vi "Generate Waveform.vi"(0 "signal configuration":refnum<class "SV Continuous Sweep.lvclass">, 5 "template waveform":waveform(dbl), 9 "samples":i32, 11 "error in (no error)":errorcluster) -> (4 "signal configuration":refnum<class "SV Continuous Sweep.lvclass">, 6 "chirp waveform":waveform(dbl), 10 "samples":i32, 15 "error out":errorcluster)   [LabVIEW 2017, in "SV Continuous Sweep.lvclass"]
uses:
  <vilib>/addons/_NISVFA/_Generation/Signal Generation/SV Continuous Sweep/SV Continuous Sweep.lvclass
  C:/Program Files (x86)/National Instruments/LabVIEW 2017/vi.lib/addons/_NISVFA/_Generation/Signal Generation/SV Signal/SV Signal.lvclass
  <vilib>/addons/_NISVFA/_Generation/Signal Generation/SV Continuous Sweep/SV Continuous Sweep.lvclass/SV Continuous Sweep.ctl
  <vilib>/addons/_NISVFA/_Generation/Signal Generation/SV Signal/sv_Signal State Attribute.ctl
  <vilib>/addons/_NISVFA/_Generation/subVIs/sv_Chirp Settings.ctl
  <vilib>/Analysis/1siggen.llb/Ramp Pattern.vi
  <vilib>/Analysis/1siggen.llb/Ramp Pattern by Samples.vi
  <vilib>/addons/_NISVFA/_Generation/Signal Generation/SV Signal/Read Sample Rate.vi
  <vilib>/addons/_NISVFA/_Generation/Signal Generation/SV Signal/SV Signal.lvclass
  <vilib>/addons/_NISVFA/_Generation/SoundVib_Generation.lvlib
  <vilib>/measure/NI_MABase.lvlib
  <vilib>/Analysis/NI_AALBase.lvlib
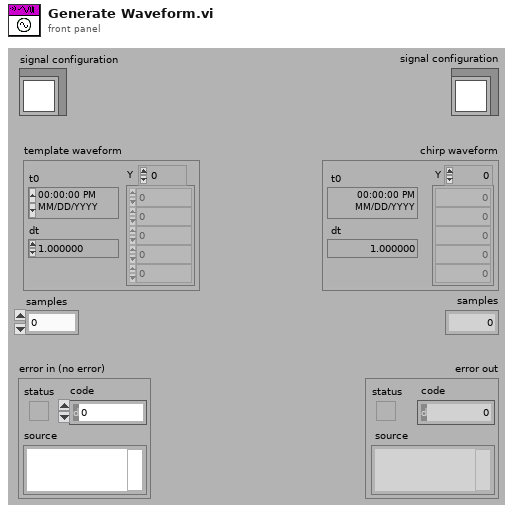
[diagram p1: front panel]
types:
  T1 = cluster{"frequency [Hz]":dbl, "phase [rad]":dbl, "elapsed time [s]":dbl}
  T2 = typedef "SoundVib_Generation.lvlib/sv_Chirp Settings.ctl" = cluster{"amplitude":dbl, "frequency range":cluster{"start (Hz)":dbl, "stop (Hz)":dbl, "frequency spacing":enum16{"Linear", "Logarithmic"}}, "sampling info":cluster{"Fs":dbl, "chirp duration [s]":dbl}, "initial states":cluster{"frequency [Hz]":dbl, "phase [rad]":dbl, "elapsed time [s]":dbl}, "frequency slope":dbl, "maximum harmonic":i32, "prefix len [samples]":cluster{"integer":u32, "fractional":dbl}}
  T3 = typedef "SV Signal.lvclass/sv_System Timing Model.ctl" = i64
  T4 = typedef "SV Signal.lvclass/sv_Generation State.ctl" = enum16{"Idle", "Ramp Up", "Pre-Measurement Settling", "Measurement", "Post-Measurement Settling", "Discrete Sweep Transition", "Ramp Down", "Update"}
  T5 = cluster{"system timing model":T3, "state":cluster{"RESET":bool, "generator timestamp":timestamp, "elapsed seconds":dbl, "elapsed samples":u64, "generation state":T4, "time offset at state":dbl, "samples generated at state":u64, "signal state":variant}, "duration of state":dbl, "samples remaining at state":i32}
  T6 = typedef "SV Signal.lvclass/sv_Signal State Attribute.ctl" = string
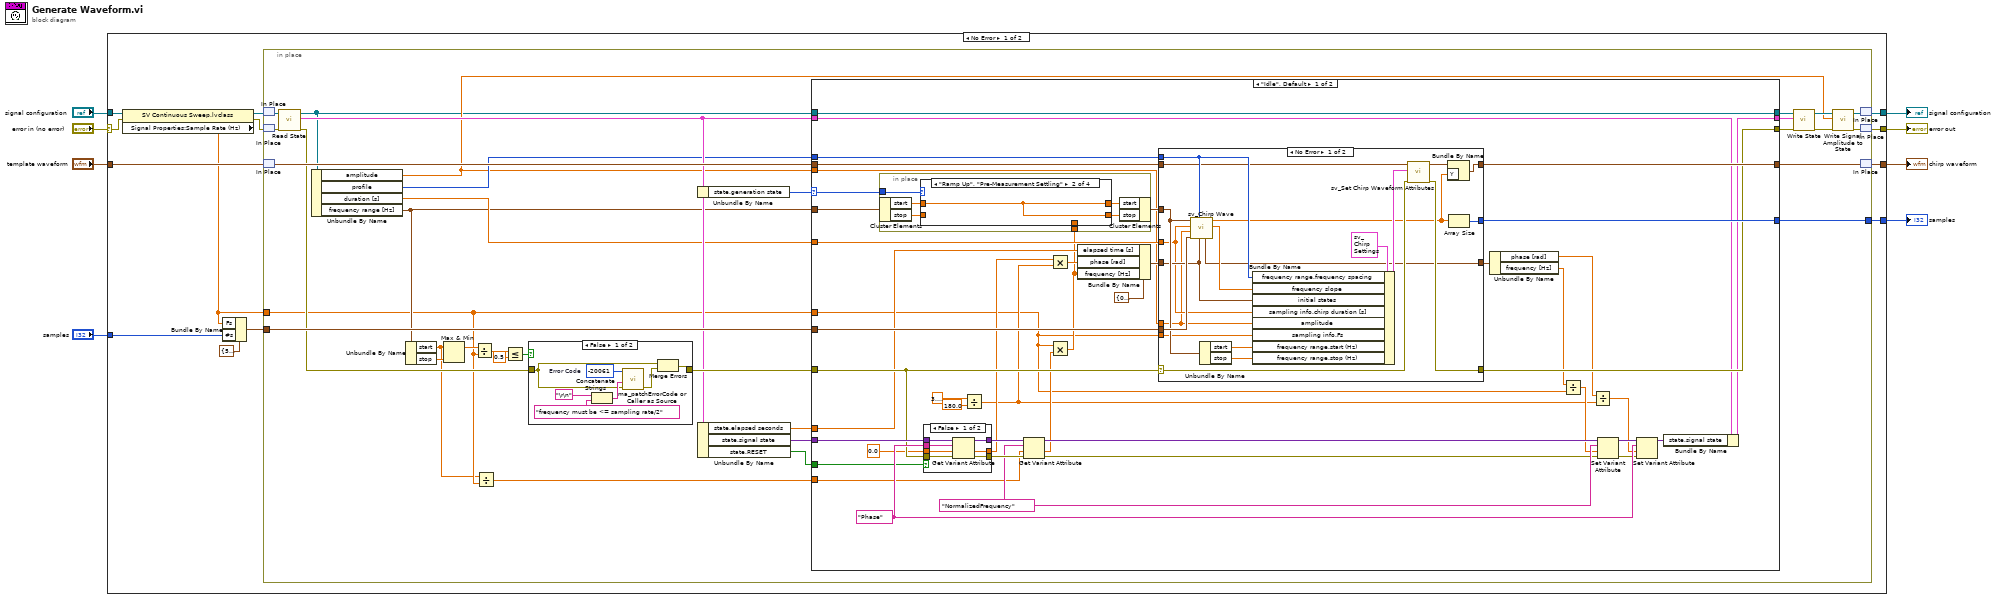
[diagram p0: block diagram]
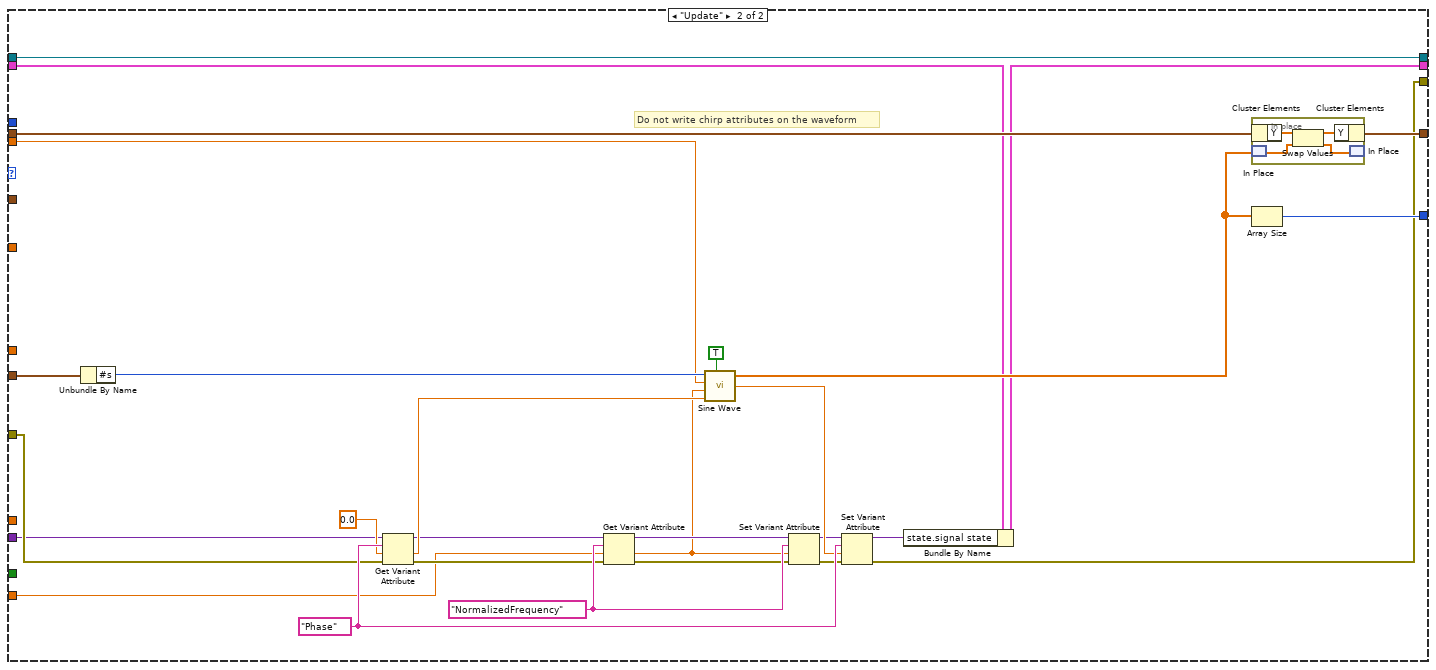
[diagram p7: hidden frame]
diagram:
  n1 = case shown="No Error" "error in (no error)" {
    selector: "error in (no error)" -> [w10 w185]
    tunnel: [w13 w185] -> w7
    tunnel: [w16 w184] -> w5
    tunnel: "signal configuration" -> [w19 w184]
    tunnel: [w14 w183] -> w4
    tunnel: "samples" -> [w20 _]
    tunnel: "template waveform" -> [w15 w183]
    tunnel: [w12 _] -> w1
    frame No Error {
      n2 = property class="SV Continuous Sweep.lvclass"(reference=w19, error in=w10) -> (reference out=w17:refnum<class "SV Continuous Sweep.lvclass">, error out=w9:errorcluster, "Signal Properties:Sample Rate (Hz)"=w11:dbl)
      n3 = Bundle By Name(cluster=cluster{"Fs":dbl, "#s":u32} {"Fs"=51200.0, "#s"=1024} ("sampling info"), "Fs"=w11, "#s"=w20) -> (w18:cluster{"Fs":dbl, "#s":u32})
      n4 = in-place {
        in-place-border: w18 -> [w47]
        in-place-border: [w48] -> w12
        in-place-border: w11 -> [w24]
        n5 = in-place-match #1(w17) -> (w43:refnum<class "SV Continuous Sweep.lvclass">)
        n6 = in-place-match #2(w9) -> (w42:errorcluster)
        n7 = in-place-match #3(w15) -> (w46:waveform(dbl))
        n8 = call <vilib>:"Read State.vi"("error in (no error)"=w42, "signal configuration"=w43) -> ("error out"=w41:errorcluster, "generator state"=w33:T5, "signal configuration"=w27:refnum<class "SV Continuous Sweep.lvclass">)  [unwired: 7 in]
        n9 = Unbundle By Name(w27) -> ("amplitude"=w29:dbl, "profile"=w30:u16, "duration [s]"=w32:dbl, "frequency range [Hz]"=w31:cluster{"start":dbl, "stop":dbl})
        n10 = Unbundle By Name(w31) -> ("start"=w23:dbl, "stop"=w52:dbl)
        n11 = Max & Min(x=w23, y=w52) -> (max(x,y)=w49:dbl)  [unwired: 1 out]
        n12 = Divide(x=w49, y=w24) -> (x/y=w51:dbl)
        n13 = Divide(x=w23, y=w24) -> (x/y=w22:dbl)
        n14 = Less Or Equal?(x=w51, y=0.5) -> (x <= y?=w35:bool)
        n15 = case shown="False" w35 {
          tunnel: [w175 w182] -> w40
          tunnel: w41 -> [w177 w182]
          frame False {
            w178 = -20061  # Error Code
            n16 = Concatenate Strings("\r\n", "frequency must be <= sampling rate/2" ("freq error message")) -> (w181:string)
            n17 = call <vilib>:"ma_patchErrorCode or Caller as Source.vi"("error in (no error)"=w177, "string to append to source"=w181, "error code"=w178) -> ("error out"=w176:errorcluster)  [unwired: 8 in]
            n18 = Merge Errors(w177, w176) -> (w175:errorcluster)
          }
          frame True {
          }
        }
        n19 = Unbundle By Name(w33) -> ("state.generation state"=w28:T4)
        n20 = Unbundle By Name(w33) -> ("state.elapsed seconds"=w34:dbl, "state.signal state"=w44:variant, "state.RESET"=w25:bool)
        n21 = case shown="\"Idle\", Default" w28 {
          selector: w28 -> [w60 _]
          tunnel: [w96 w162] -> w48
          tunnel: w47 -> [w95 w160]
          tunnel: w46 -> [w93 w161]
          tunnel: [w92 w163] -> w45
          tunnel: w44 -> [w87 w166]
          tunnel: w25 -> [w86 _]
          tunnel: w40 -> [w85 w167]
          tunnel: [w84 w152] -> w37
          tunnel: [w83 w154] -> w36
          tunnel: w34 -> [w76 _]
          tunnel: w24 -> [w57 _]
          tunnel: w33 -> [w66 w155]
          tunnel: w32 -> [w64 _]
          tunnel: w31 -> [w56 _]
          tunnel: w30 -> [w63 _]
          tunnel: w29 -> [w61 w158]
          tunnel: w27 -> [w59 w153]
          tunnel: [w59 w153] -> w26
          tunnel: w22 -> [w55 w143]
          frame "Idle", Default {
            w88 = T6 "Phase" ("name")
            w79 = T6 "NormalizedFrequency" ("name")
            n22 = case shown="False" w86 {
              tunnel: w87 -> [w116 w118]
              tunnel: 0.0 ("phase in [deg]") -> [w115 w119]
              tunnel: [w114 w119] -> w82
              tunnel: [w113 w118] -> w90
              tunnel: w85 -> [w112 w117]
              tunnel: [w111 w117] -> w89
              tunnel: w88 -> [w110 _]
              frame False {
                n23 = Get Variant Attribute(Variant=w116, name=w110, default value (empty Variant)=w115, error in=w112) -> (duplicate Variant=w113:variant, value=w114:dbl, error out=w111:errorcluster)  [unwired: 1 out]
              }
              frame True {
              }
            }
            n24 = Divide(x=3.141592653589793, y=180.0 ("value")) -> (x/y=w68:dbl)
            n25 = Get Variant Attribute(Variant=w90, name=w79, default value (empty Variant)=w55, error in=w89) -> (duplicate Variant=w78:variant, value=w75:dbl, error out=w77:errorcluster)  [unwired: 1 out]
            n26 = Multiply(x=w82, y=w68) -> (x*y=w97:dbl)
            n27 = Multiply(x=w57, y=w75) -> (x*y=w58:dbl)
            n28 = in-place {
              in-place-border: w60 -> [w104]
              in-place-border: w58 -> [w99]
              n29 = in-place-cluster #4(w56) -> ("start"=w103:dbl, "stop"=w102:dbl)
              n30 = case shown="\"Ramp Up\", \"Pre-Measurement Settling\"" w104 {
                tunnel: w103 -> [w106 w107 _ _]
                tunnel: w102 -> [w105 _ w108 _]
                tunnel: [w106 w107 w108 w109] -> w101
                tunnel: [w105 w107 w108 w109] -> w100
                tunnel: w99 -> [_ _ _ w109]
                frame "Idle", "Measurement", Default {
                }
                frame "Ramp Up", "Pre-Measurement Settling" {
                }
                frame "Post-Measurement Settling" {
                }
                frame "Ramp Down" {
                }
              }
              n31 = in-place-cluster #4("start"=w101, "stop"=w100) -> (w65:cluster{"start":dbl, "stop":dbl})
            }
            n32 = Bundle By Name(cluster=T1 {"frequency [Hz]"=0.0, "phase [rad]"=0.0, "elapsed time [s]"=0.0} ("initial states"), "elapsed time [s]"=w76, "phase [rad]"=w97, "frequency [Hz]"=w58) -> (w94:T1)
            n33 = case shown="No Error" w85 {
              selector: w85 -> [w139 w142]
              tunnel: w95 -> [w136 _]
              tunnel: w65 -> [w135 _]
              tunnel: w64 -> [w123 _]
              tunnel: w61 -> [w122 _]
              tunnel: [w137 w142] -> w84
              tunnel: [w138 w141] -> w92
              tunnel: w63 -> [w134 _]
              tunnel: w93 -> [w133 w141]
              tunnel: [w132 _] -> w96
              tunnel: w94 -> [w131 w140]
              tunnel: w57 -> [w121 _]
              tunnel: [w120 w140] -> w73
              frame No Error {
                n34 = call <vilib>:"sv_Chirp Wave.vi"("state in"=w131, "frequency spacing"=w134, "sampling info"=w136, "amplitude"=w122, "chirp duration [s]"=w123, "frequency range"=w135) -> ("frequency slope"=w125:dbl, "chirp wave"=w124:dbl[], "state out"=w120:T1)  [unwired: 3 in]
                n35 = Unbundle By Name(w135) -> ("start"=w127:dbl, "stop"=w126:dbl)
                n36 = Bundle By Name(cluster=T2 {"amplitude"=1.0, "frequency range"={"start (Hz)"=20.0, "stop (Hz)"=20000.0, "frequency spacing"=enum."Logarithmic"}, "sampling info"={"Fs"=50000.0, "chirp duration [s]"=3.0}, "initial states"={"frequency [Hz]"=20.0, "phase [rad]"=0.0, "elapsed time [s]"=0.0}, "frequency slope"=0.0, "maximum harmonic"=3, "prefix len [samples]"={"integer"=0, "fractional"=0.0}} ("chirp settings"), "frequency range.frequency spacing"=w134, "frequency slope"=w125, "initial states"=w131, "sampling info.chirp duration [s]"=w123, "amplitude"=w122, "sampling info.Fs"=w121, "frequency range.start (Hz)"=w127, "frequency range.stop (Hz)"=w126) -> (w129:T2)
                n37 = call <vilib>:"sv_Set Chirp Waveform Attributes.vi"("error in (no error)"=w139, "chirp settings"=w129, "chirp signal"=w133) -> ("error out"=w137:errorcluster, "chirp signal out"=w128:waveform(dbl))  [unwired: 7 in]
                n38 = Bundle By Name(cluster=w128, "Y"=w124) -> (w138:waveform(dbl))
                n39 = Array Size(array=w124) -> (size(s)=w132:i32)
              }
              frame Error {
              }
            }
            n40 = Unbundle By Name(w73) -> ("phase [rad]"=w69:dbl, "frequency [Hz]"=w74:dbl)
            n41 = Divide(x=w74, y=w57) -> (x/y=w72:dbl)
            n42 = Divide(x=w69, y=w68) -> (x/y=w67:dbl)
            n43 = Set Variant Attribute(Variant=w78, name=w79, value=w72, error in=w77) -> (Variant out=w81:variant, error out=w80:errorcluster)  [unwired: 1 out]
            n44 = Set Variant Attribute(Variant=w81, name=w88, value=w67, error in=w80) -> (Variant out=w91:variant)  [unwired: 2 out]
            n45 = Bundle By Name(cluster=w66, "state.signal state"=w91) -> (w83:T5)
          }
          frame "Update" {
            w169 = T6 "Phase" ("name")
            w151 = T6 "NormalizedFrequency" ("name")
            # "Do not write chirp attributes on the waveform"
            n46 = Unbundle By Name(w160) -> ("#s"=w159:u32)
            n47 = Get Variant Attribute(Variant=w166, name=w169, default value (empty Variant)=0.0 ("phase in [deg]"), error in=w167) -> (duplicate Variant=w145:variant, value=w157:dbl, error out=w144:errorcluster)  [unwired: 1 out]
            n48 = Get Variant Attribute(Variant=w145, name=w151, default value (empty Variant)=w143, error in=w144) -> (duplicate Variant=w147:variant, value=w146:dbl, error out=w148:errorcluster)  [unwired: 1 out]
            n49 = call <vilib>:"Sine Wave.vi"("samples"=w159, "amplitude"=w158, "frequency"=w146, "phase in"=w157, "reset phase"=TRUE) -> ("sine wave"=w164:dbl[], "phase out"=w156:dbl)  [unwired: 1 out]
            n50 = Set Variant Attribute(Variant=w147, name=w151, value=w146, error in=w148) -> (Variant out=w149:variant, error out=w150:errorcluster)  [unwired: 1 out]
            n51 = Set Variant Attribute(Variant=w149, name=w169, value=w156, error in=w150) -> (Variant out=w170:variant, error out=w152:errorcluster)  [unwired: 1 out]
            n52 = Bundle By Name(cluster=w155, "state.signal state"=w170) -> (w154:T5)
            n53 = in-place {
              n54 = in-place-cluster #5(w161) -> ("Y"=w174:dbl[])
              n55 = in-place-match #6(w164) -> (w172:dbl[])
              n56 = Swap Values(12:w174, 14:w172) -> (1:w173:dbl[], 3:w171:dbl[])  [unwired: 1 in]
              n57 = in-place-cluster #5("Y"=w173) -> (w163:waveform(dbl))
              n58 = in-place-match #6(w171) -> ()  [unwired: 1 out]
            }
            n59 = Array Size(array=w164) -> (size(s)=w162:i32)
          }
        }
        n60 = call <vilib>:"Write State.vi"("error in (no error)"=w37, "generator state"=w36, "signal configuration"=w26) -> ("error out"=w38:errorcluster, "signal configuration"=w39:refnum<class "SV Continuous Sweep.lvclass">)  [unwired: 7 in]
        n61 = call <vilib>:"Write Signal Amplitude to State.vi"("error in (no error)"=w38, "amplitude"=w29, "SV Signal in"=w39) -> ("error out"=w53:errorcluster, "SV Signal out"=w54:refnum<class "SV Continuous Sweep.lvclass">)  [unwired: 7 in]
        n62 = in-place-match #1(w54) -> (w16:refnum<class "SV Continuous Sweep.lvclass">)
        n63 = in-place-match #2(w53) -> (w13:errorcluster)
        n64 = in-place-match #3(w45) -> (w14:waveform(dbl))
      }
    }
    frame Error {
    }
  }
  "error out" <- w7
  "signal configuration" <- w5
  "chirp waveform" <- w4
  "samples" <- w1
